vi "determine execution settings.vi"(11 "channels":refnum<class "TBM channel.lvclass">[](array[class])) -> (3 "execution settings":T1)   [LabVIEW 2013, in "TBM module execution interface.lvclass"]
doc: "Converts a list of channels into the execution settings for the configuration. This may be used by modules to simplify the configuration process. The execution settings will be set true if any channel provided matches that execution setting."
uses:
  TBM module execution interface.lvclass
  channel/TBM channel.lvclass
  execution settings.ctl
  channel/TBM channel.lvclass/TBM channel.ctl
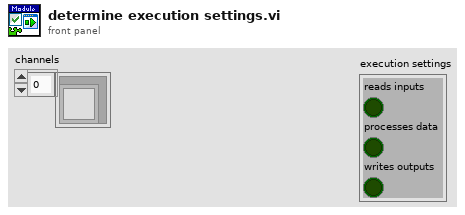
[diagram p1: front panel]
types:
  T1 = typedef "TBM module execution interface.lvclass/execution settings.ctl" = cluster{"reads inputs":bool, "processes data":bool, "writes outputs":bool}
  T2 = typedef "TBM channel.lvclass/channel classification.ctl" = enum16{"input data", "output data", "processing parameter", "processing result"}
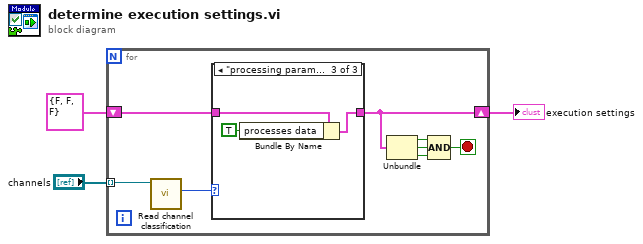
[diagram p0: block diagram]
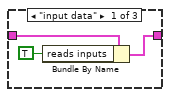
[diagram p2: hidden frame]
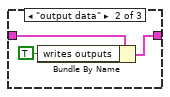
[diagram p3: hidden frame]
diagram:
  n1 = for {
    tunnel: "channels" -> [w11] mode=indexing
    shift-right: [w8] -> w1
    shift-left: T1 {"reads inputs"=FALSE, "processes data"=FALSE, "writes outputs"=FALSE} ("execution settings") -> [w9]
    stop <- w4 stop-if-true
    n2 = call "Read channel classification.vi"("channel in"=w11) -> ("channel classification"=w10:T2)  [unwired: 8 in, 2 out]
    n3 = case shown="\"processing parameter\", Default" w10 {
      tunnel: w9 -> [w14 w17 w20]
      tunnel: [w12 w15 w18] -> w8
      frame "input data" {
        n4 = Bundle By Name(cluster=w14, "reads inputs"=TRUE) -> (w12:T1)
      }
      frame "output data" {
        n5 = Bundle By Name(cluster=w17, "writes outputs"=TRUE ("reads inputs")) -> (w15:T1)
      }
      frame "processing parameter", Default {
        n6 = Bundle By Name(cluster=w20, "processes data"=TRUE ("reads inputs")) -> (w18:T1)
      }
    }
    n7 = Unbundle(w8) -> ("reads inputs"=w5:bool, "processes data"=w6:bool, "writes outputs"=w7:bool)
    n8 = Compound Arithmetic op=AND(w5, w6, w7) -> (w4:bool)
  }
  "execution settings" <- w1
